vi "Test_ChainedCalls.vi"() -> ()   [LabVIEW 2019]
uses:
  FetchCalibration/Converted_Slug_Cluster.ctl
  <vilib>/Bytelabs/ByteREST/CfgLoaders/LoaderBase/ServerParams.ctl
  <vilib>/Bytelabs/ByteREST/ByteRESTClass/ByteRESTBase/Auth/Authentication_type.ctl
  CalibrationMeasurements/BodyCalibrazioneMisure.ctl
  ByteGSAPIBase.lvclass
  <vilib>/Bytelabs/ByteREST/ByteRESTClass/ByteRESTBase/RESTBase.lvclass
  <vilib>/Bytelabs/ByteREST/CfgLoaders/LoaderBase/RESTLoaderBase.lvclass
panel:
  in  "instrument measure":sgl
  in  "measurement id":u16
  out "measurements":cluster{"id":u32, "passed":bool}[](array[cluster])
  out "measurement_group_passed":bool
  out "Calibration data":T1 {"controls"."umidita" format="%.1g"; "controls"."temperatura_c" format="%.1g"; "controls"."incertezza" format="%.1g"; "controls"."deviazione_standard" format="%.1g"; "controls"."mpe_min" format="%.1g"; "controls"."mpe_max" format="%.1g"; "controls"."riferimento_obiettivo" format="%.1g"}
  in  "Server cfg":T2={"API Root"="", "verify server"=FALSE, "Version (no version)"="", "Port (protocol specific)"=0, "Base URL"="", "Auth type"=enum."Token", "Auth string"="", "timeout (10000)"=10000}
  out "Instruments out":T4[](array[typedef])
  out "error out":errorcluster
  in  "Instruments":string[](array[string])
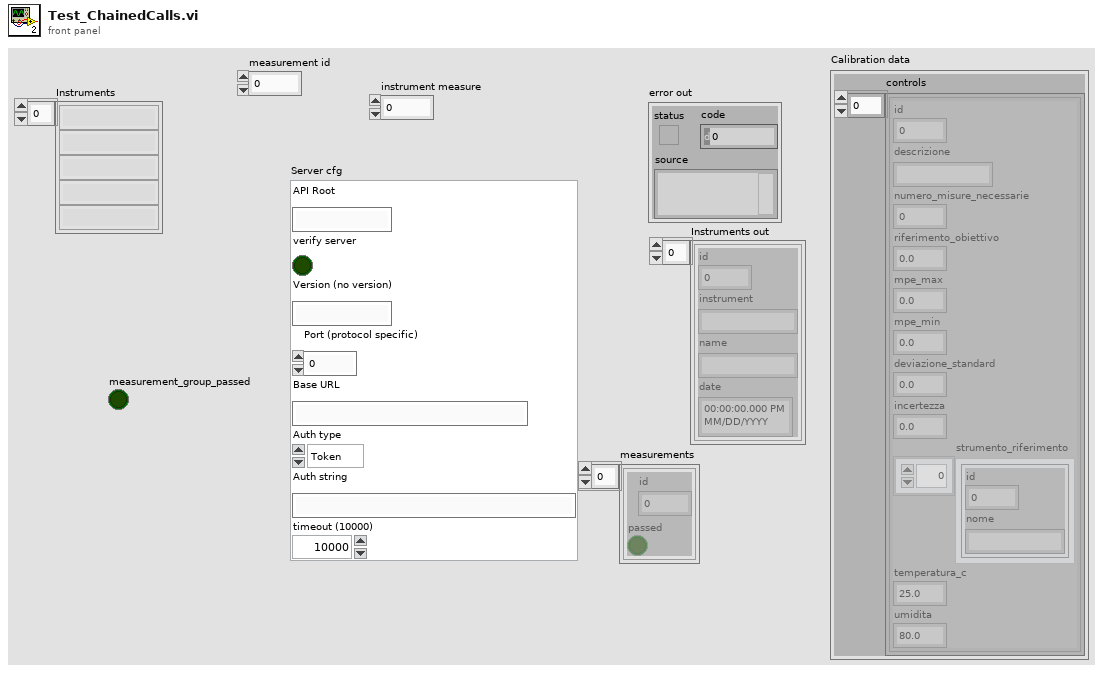
[diagram p1: front panel]
types:
  T1 = typedef "ByteGSWebAPI.lvlib/ByteGSAPIBase.lvclass/BodyCalibrazioneMisure.ctl" = cluster{"controls":cluster{"id":u16, "descrizione":string, "numero_misure_necessarie":u16, "riferimento_obiettivo":dbl, "mpe_max":dbl, "mpe_min":dbl, "deviazione_standard":dbl, "incertezza":dbl, "strumento_riferimento":cluster{"id":u16, "nome":string}[], "temperatura_c":dbl, "umidita":dbl}[]}
  T2 = typedef "ByteREST.lvlib/RESTLoaderBase.lvclass/ServerParams.ctl" = cluster{"API Root":string, "verify server":bool, "Version (no version)":string, "Port (protocol specific)":u16, "Base URL":string, "Auth type":T3, "Auth string":string, "timeout (10000)":i32}
  T3 = typedef "ByteREST.lvlib/RESTBase.lvclass/Authentication_type.ctl" = enum16{"Token"}
  T4 = typedef "ByteGSWebAPI.lvlib/ByteGSAPIBase.lvclass/Converted_Slug_Cluster.ctl" = cluster{"id":u32, "instrument":string, "name":string, "date":timestamp}
  T5 = cluster{"id":u16, "descrizione":string, "numero_misure_necessarie":u16, "riferimento_obiettivo":dbl, "mpe_max":dbl, "mpe_min":dbl, "deviazione_standard":dbl, "incertezza":dbl, "strumento_riferimento":cluster{"id":u16, "nome":string}[], "temperatura_c":dbl, "umidita":dbl}[]
  T6 = cluster{"id":u16, "descrizione":string, "numero_misure_necessarie":u16, "riferimento_obiettivo":dbl, "mpe_max":dbl, "mpe_min":dbl, "deviazione_standard":dbl, "incertezza":dbl, "strumento_riferimento":cluster{"id":u16, "nome":string}[], "temperatura_c":dbl, "umidita":dbl}
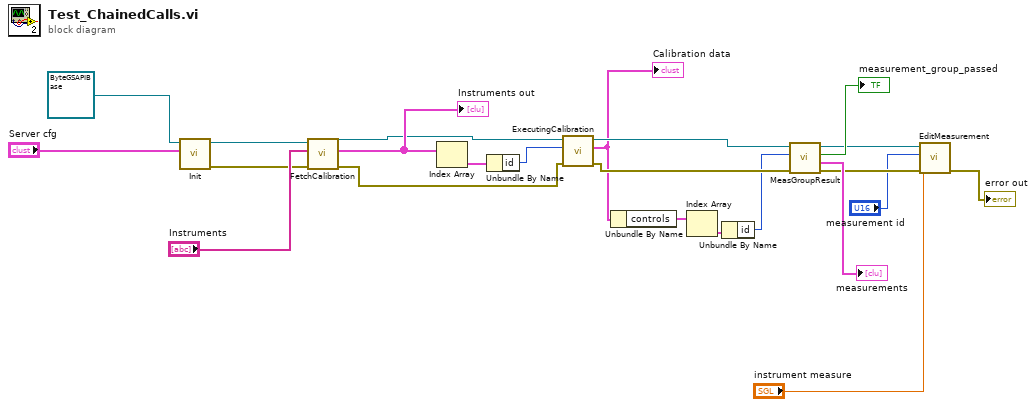
[diagram p0: block diagram]
diagram:
  n1 = call-dynamic "Init.vi"("Server cfg"="Server cfg", "ByteGSAPIBase in"=refnum<class "ByteGSAPIBase.lvclass"> refnum) -> ("error out"=w20:errorcluster, "ByteGSAPIBase out"=w21:refnum<class "ByteGSAPIBase.lvclass">)  [unwired: 8 in]
  n2 = call "FetchCalibration.vi"("error in (no error)"=w20, "Instruments"="Instruments", "ByteGSAPIBase in"=w21) -> ("error out"=w14:errorcluster, "Instruments"=w18:T4[], "ByteGSAPIBase out"=w16:refnum<class "ByteGSAPIBase.lvclass">)  [unwired: 6 in]
  "Instruments out" <- w18
  n3 = Index Array(array=w18) -> (element=w17:T4)  [unwired: 1 in]
  n4 = Unbundle By Name(w17) -> ("id"=w15:u32)
  n5 = call "ExecutingCalibration.vi"("error in (no error)"=w14, "calibration_id"=w15, "ByteGSAPIBase in"=w16) -> ("error out"=w12:errorcluster, "Calibration data"=w6:T1, "ByteGSAPIBase out"=w13:refnum<class "ByteGSAPIBase.lvclass">)  [unwired: 6 in]
  "Calibration data" <- w6
  n6 = Unbundle By Name(w6) -> ("controls"=w5:T5)
  n7 = Index Array(array=w5) -> (element=w4:T6)  [unwired: 1 in]
  n8 = Unbundle By Name(w4) -> ("id"=w3:u16)
  n9 = call "MeasGroupResult.vi"("error in (no error)"=w12, "measurement_group_id"=w3, "ByteGSAPIBase in"=w13) -> ("error out"=w7:errorcluster, "measurements"=→"measurements":cluster{"id":u32, "passed":bool}[], "measurement_group_passed"=→"measurement_group_passed":bool, "ByteGSAPIBase out"=w9:refnum<class "ByteGSAPIBase.lvclass">)  [unwired: 5 in]
  n10 = call-dynamic "EditMeasurement.vi"("error in (no error)"=w7, "instrument measure"="instrument measure", "measurement id"="measurement id", "ByteGSAPIBase in"=w9) -> ("error out"=→"error out":errorcluster)  [unwired: 4 in, 3 out]
